vi "VI Tree_Image Processing.vi"   [LabVIEW 2014]
panel:
  # "See Block Diagram"
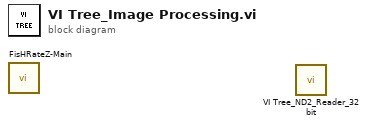
[diagram p0: block diagram]
diagram:
  n1 = call "FisHRateZ-Main.vi"() -> ()  [unwired: 12 in]
  n2 = call "VI Tree_ND2_Reader_32 bit.vi"() -> ()  [unwired: 12 in]
